vi "CheckForWinDeath.vi"(8 "error in (no error)":errorcluster, 11 "Bouncer in":refnum<class "Bouncer.lvclass">) -> (0 "error out":errorcluster, 3 "Bouncer out":refnum<class "Bouncer.lvclass">)   [LabVIEW 2019, in "RT_Game.lvlib" / "Bouncer.lvclass"]
uses:
  Bouncer.lvclass
  C:/Users/FreshBob/Dropbox/VIs/myRIO_GameConsole/RT/RT_Game/Game/Game.lvclass
  Bouncer.lvclass/Bouncer.ctl
  GameObject/GameObject.lvclass/GameObject.ctl
  GameObject/Read IsActive.vi
  GameObject/Read position.vi
  BounceTarget/BounceTarget.lvclass
  C:/Users/FreshBob/Dropbox/VIs/myRIO_GameConsole/RT/RT_Game/GameObject/GameObject.lvclass
  PongBall/PongBall.lvclass
  Game/Game.lvclass
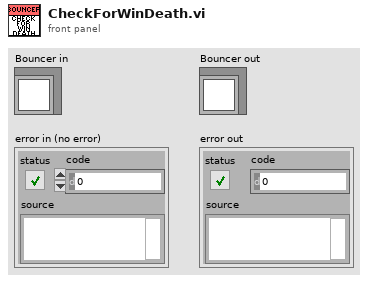
[diagram p1: front panel]
types:
  T1 = typedef "RT_Game.lvlib/Game.lvclass/Coordinate.ctl" = cluster{"x":dbl, "y":dbl}
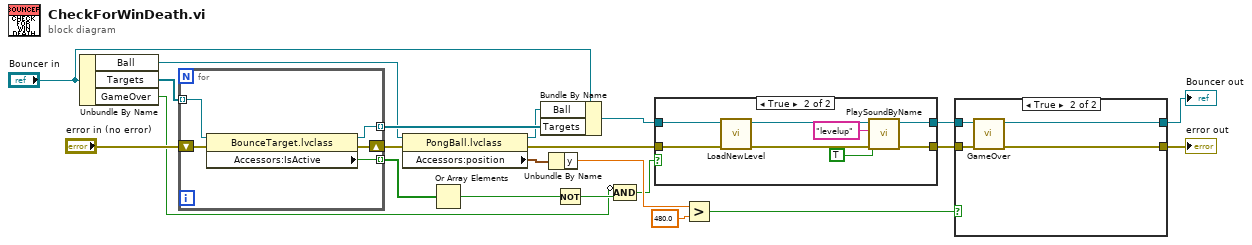
[diagram p0: block diagram]
diagram:
  n1 = Unbundle By Name("Bouncer in") -> ("Ball"=w15:refnum<class "PongBall.lvclass">, "Targets"=w19:refnum<class "BounceTarget.lvclass">[], "GameOver"=w1:bool)
  n2 = for {
    tunnel: w19 -> [w25] mode=indexing
    tunnel: [w24] -> w18 mode=indexing
    shift-right: [w26] -> w20
    shift-left: "error in (no error)" -> [w27]
    tunnel: [w23] -> w17 mode=indexing
    n3 = property class="BounceTarget.lvclass"(reference=w25, error in=w27) -> (reference out=w24:refnum<class "BounceTarget.lvclass">, error out=w26:errorcluster, "Accessors:IsActive"=w23:bool)
  }
  n4 = property class="PongBall.lvclass"(reference=w15, error in=w20) -> (reference out=w14:refnum<class "PongBall.lvclass">, error out=w5:errorcluster, "Accessors:position"=w13:T1)
  n5 = Or Array Elements(Boolean array=w17) -> (logical OR=w16:bool)
  n6 = Bundle By Name(cluster="Bouncer in", "Ball"=w14, "Targets"=w18) -> (w7:refnum<class "Bouncer.lvclass">)
  n7 = Unbundle By Name(w13) -> ("y"=w12:dbl)
  n8 = Not(x=w16) -> (.not. x?=w3:bool)
  n9 = Compound Arithmetic op=AND(invert w1, w3) -> (w2:bool)
  n10 = case shown="True" w2 {
    tunnel: w7 -> [w28 w35]
    tunnel: [w28 w32] -> w6
    tunnel: [w29 w34] -> w4
    tunnel: w5 -> [w29 w37]
    frame False {
    }
    frame True {
      n11 = call "LoadNewLevel.vi"("error in (no error)"=w37, "Bouncer in"=w35) -> ("error out"=w36:errorcluster, "Bouncer out"=w33:refnum<class "Bouncer.lvclass">)  [unwired: 8 in]
      n12 = call "PlaySoundByName.vi"("error in (no error)"=w36, "Overwrite"=TRUE, "Name"="levelup", "Game in"=w33) -> ("error out"=w34:errorcluster, "Game out"=w32:refnum<class "Bouncer.lvclass">)  [unwired: 6 in]
    }
  }
  n13 = Greater?(x=w12, y=480.0) -> (0:w9:bool)
  n14 = case shown="True" w9 {
    tunnel: w6 -> [w38 w42]
    tunnel: [w38 w40] -> w8
    tunnel: [w39 w41] -> w10
    tunnel: w4 -> [w39 w43]
    frame False {
    }
    frame True {
      n15 = call "GameOver.vi"("error in (no error)"=w43, "Bouncer in"=w42) -> ("error out"=w41:errorcluster, "Bouncer out"=w40:refnum<class "Bouncer.lvclass">)  [unwired: 8 in]
    }
  }
  "error out" <- w10
  "Bouncer out" <- w8
